vi "Get ai_parameter.vi"(7 "模式":i32(slide) scale=0.0..1.0, 8 "采样速率":dbl, 9 "Sing_ch":bool[](array[boolean]), 10 "Diff_ch":bool[](array[boolean]), 11 "Device name":string="Dev01/ai") -> (2 "Daq_ai_para":T1={"Channel"=[], "Sample rate"=0.0, "input terminal configuration"=-1} {"input terminal configuration" items=["Default"=-1, "RSE"=10083, "NRSE"=10078, "Differential"=10106, "Pseudodifferential"=12529]})   [LabVIEW 2017]
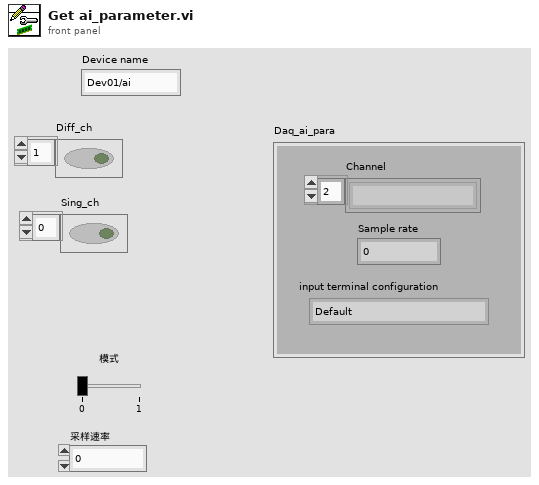
[diagram p1: front panel]
types:
  T1 = cluster{"Channel":string[], "Sample rate":dbl, "input terminal configuration":i32}
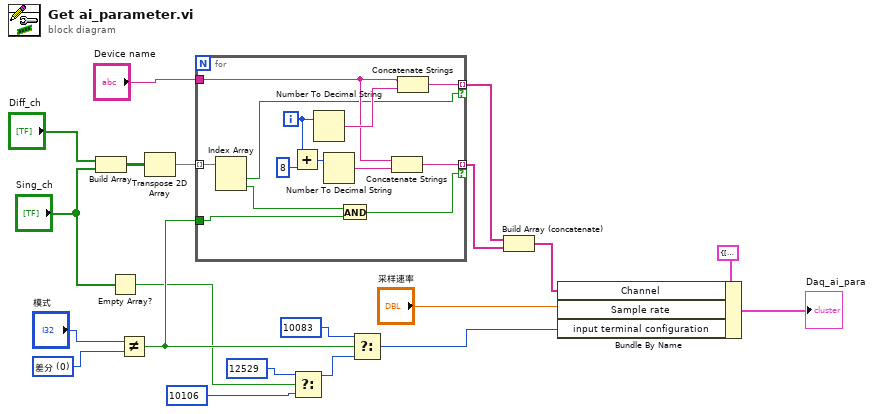
[diagram p0: block diagram]
diagram:
  w16 = 0 items=["差分", "单端"] ("模式")
  n1 = Build Array("Diff_ch", "Sing_ch") -> (w7:bool[][])
  n2 = Empty Array?(array="Sing_ch") -> (empty?=w2:bool)
  n3 = Not Equal?(x="模式", y=w16) -> (x != y?=w13:bool)
  n4 = Transpose 2D Array(2D array=w7) -> (transposed array=w6:bool[][])
  n5 = for {
    tunnel: w13 -> [w25]
    tunnel: "Device name" -> [w29]
    tunnel: [w27] -> w11 mode=indexing if=w22
    tunnel: [w26] -> w10 mode=indexing if=w24
    tunnel: w6 -> [w23] mode=indexing
    i -> [w32]
    n6 = Index Array(array=w23) -> (element #1=w22:bool, element #2=w21:bool)  [unwired: 2 in]
    n7 = Add(x=w32, y=8) -> (x+y=w31:i32)
    n8 = Number To Decimal String(number=w32) -> (decimal integer string=w33:string)  [unwired: 1 in]
    n9 = Number To Decimal String(number=w31) -> (decimal integer string=w28:string)  [unwired: 1 in]
    n10 = And(x=w21, y=w25) -> (x .and. y?=w24:bool)
    n11 = Concatenate Strings(w29, w28) -> (w26:string)
    n12 = Concatenate Strings(w29, w33) -> (w27:string)
  }
  n13 = Select(t=12529, s=w2, f=10106) -> (s? t:f=w4:i32)
  n14 = Select(t=10083 ("input terminal configuration"), s=w13, f=w4) -> (s? t:f=w14:i32)
  n15 = Build Array (concatenate)(w11, w10) -> (w9:string[])
  n16 = Bundle By Name(cluster=T1 {"Channel"=[], "Sample rate"=0.0, "input terminal configuration"=10106} ("Daq_ai_para"), "Channel"=w9, "Sample rate"="采样速率", "input terminal configuration"=w14) -> (→"Daq_ai_para":T1)
